vi "Get Configuration File String.vi"(7 "section":string, 8 "error in (no error)":errorcluster, 9 "default value":string, 10 "key":string, 11 "Application Controller in":refnum<class "Application Controller.lvclass">) -> (0 "error out":errorcluster, 1 "value":string, 2 "found?":bool, 3 "Application Controller out":refnum<class "Application Controller.lvclass">)   [LabVIEW 2016, in "Application Controller.lvclass"]
uses:
  Application Controller.lvclass
  Application Controller.lvclass/Application Controller.ctl
  <vilib>/Utility/config.llb/Read Key (String).vi
  <vilib>/Utility/config.llb/NI_LVConfig.lvlib
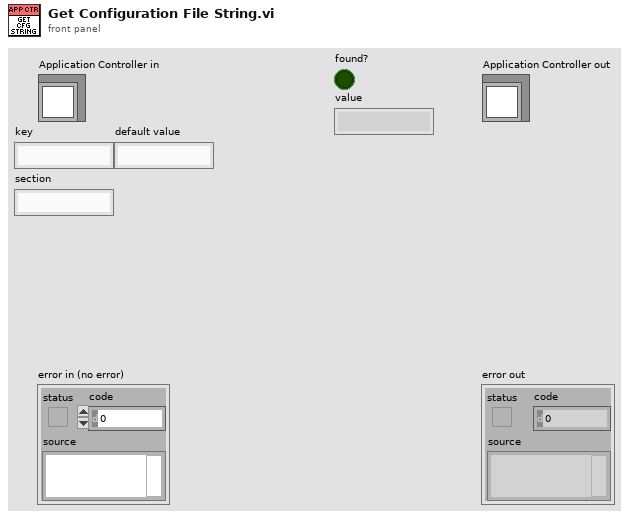
[diagram p1: front panel]
types:
  T1 = typedef "NI_LVConfig.lvlib/Config Data RefNum.ctl" = refnum<k1>
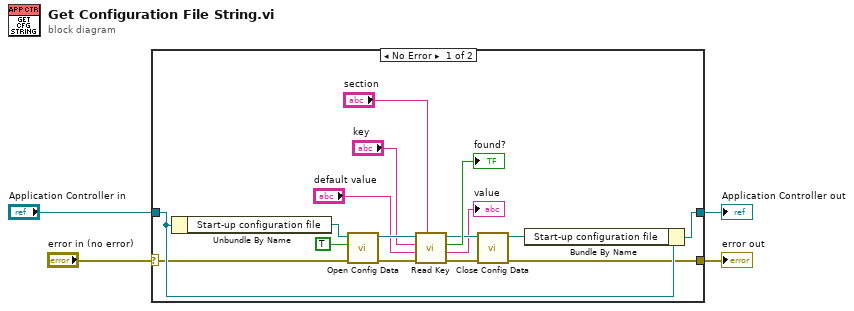
[diagram p0: block diagram]
diagram:
  n1 = case shown="No Error" "error in (no error)" {
    selector: "error in (no error)" -> [w8 w22]
    tunnel: [w7 w22] -> w3
    tunnel: [w6 w21] -> w1
    tunnel: "Application Controller in" -> [w20 w21]
    frame No Error {
      n2 = Unbundle By Name(w20) -> ("Start-up configuration file"=w19:path)
      n3 = call <vilib>:"Open Config Data.vi"("error in (no error)"=w8, "create file if necessary (T)"=TRUE, "configuration file path"=w19) -> ("error out"=w15:errorcluster, "refnum"=w17:T1)  [unwired: 6 in, 1 out]
      n4 = call-poly <vilib>:"Read Key.vi"("section"="section", "error in (no error)"=w15, "default value"="default value", "key"="key", "refnum"=w17) -> ("error out"=w10:errorcluster, "value"=→"value":string, "found?"=→"found?":bool, "refnum out"=w11:T1)  [unwired: 3 in]
      n5 = call <vilib>:"Close Config Data.vi"("error in (no error)"=w10, "refnum"=w11) -> ("error out"=w7:errorcluster, "file path"=w5:path)  [unwired: 8 in]
      n6 = Bundle By Name(cluster=w20, "Start-up configuration file"=w5) -> (w6:refnum<class "Application Controller.lvclass">)
    }
    frame Error {
    }
  }
  "error out" <- w3
  "Application Controller out" <- w1
